vi "ReadAnswer(TCS).vi"(0 "VISA resource name":refnum<visa-resource-name>, 7 "String to Send":string, 11 "Bytes to Read":u32=10, 13 "Error IN":errorcluster) -> (4 "VISA resource name dup":refnum<visa-resource-name>, 6 "String Received":string, 10 "OK Done":bool, 15 "error out":errorcluster)   [LabVIEW 2011]
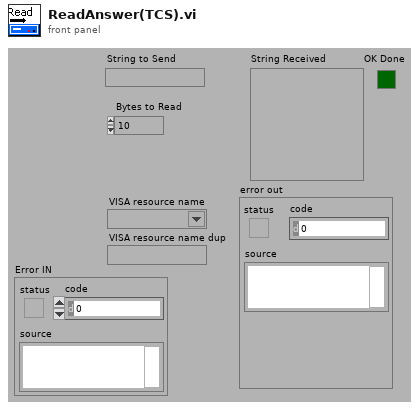
[diagram p1: front panel]
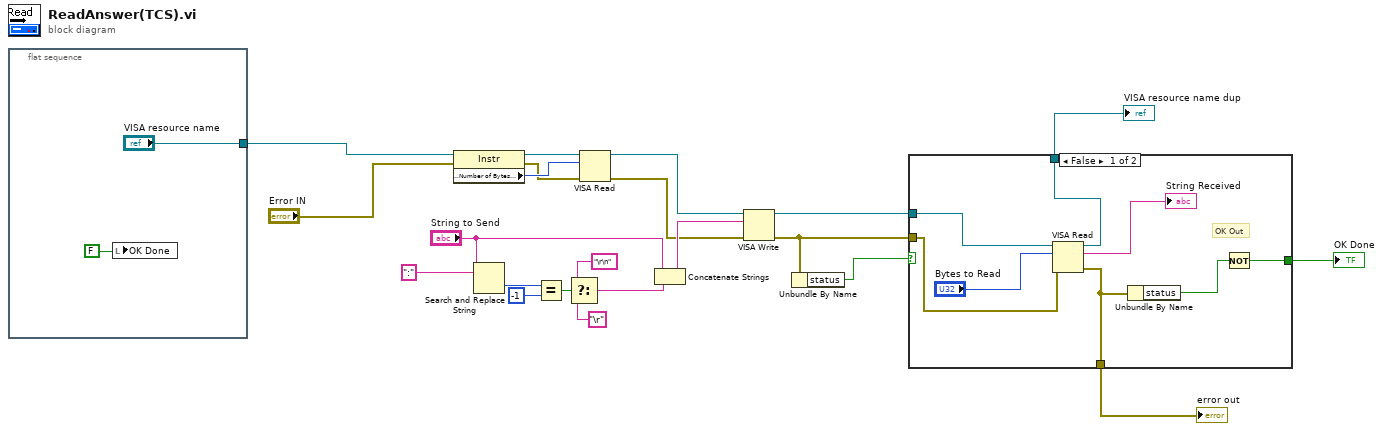
[diagram p0: block diagram]
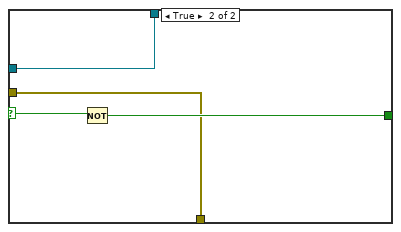
[diagram p2: hidden frame]
diagram:
  n1 = flat-sequence {
    tunnel: ["VISA resource name"] -> w10
    frame #0 {
      n2 = local write "OK Done"(FALSE) -> ()
    }
  }
  n3 = property class="Instr"(reference=w10, error in="Error IN") -> (reference out=w8:refnum<visa-resource-name>, error out=w2:errorcluster, "Serial Settings:Number of Bytes at Serial Port"=w9:u32)
  n4 = Search and Replace String(input string="String to Send", search string=":") -> (offset past replacement=w20:i32)  [unwired: 6 in, 3 out]
  n5 = Equal?(x=w20, y=-1) -> (x = y?=w18:bool)
  n6 = Select(t="\r\n", s=w18, f="\r") -> (s? t:f=w17:string)
  n7 = VISA Read(VISA resource name=w8, byte count=w9, error in (no error)=w2) -> (VISA resource name out=w7:refnum<visa-resource-name>, error out=w1:errorcluster)  [unwired: 2 out]
  n8 = Concatenate Strings("String to Send", w17) -> (w13:string)
  n9 = VISA Write(VISA resource name=w7, write buffer=w13, error in (no error)=w1) -> (VISA resource name out=w12:refnum<visa-resource-name>, error out=w4:errorcluster)  [unwired: 1 out]
  n10 = Unbundle By Name(w4) -> ("status"=w11:bool)
  n11 = case shown="False" w11 {
    selector: w11 -> [_ w36]
    tunnel: [w31 w35] -> w22
    tunnel: w12 -> [w30 w34]
    tunnel: [w27 w34] -> w6
    tunnel: [w26 w33] -> w5
    tunnel: w4 -> [w25 w33]
    frame False {
      # "OK Out"
      n12 = VISA Read(VISA resource name=w30, byte count="Bytes to Read", error in (no error)=w25) -> (VISA resource name out=w27:refnum<visa-resource-name>, read buffer=→"String Received":string, error out=w26:errorcluster)  [unwired: 1 out]
      n13 = Unbundle By Name(w26) -> ("status"=w32:bool)
      n14 = Not(x=w32) -> (.not. x?=w31:bool)
    }
    frame True {
      n15 = Not(x=w36) -> (.not. x?=w35:bool)
    }
  }
  "OK Done" <- w22
  "VISA resource name dup" <- w6
  "error out" <- w5
